vi "Read out  X Sensor.vi"() -> (1 "error out":errorcluster, 2 "Result":dbl format="%#_5p")   [LabVIEW 2013]
panel:
  # "Read Out XSensor"
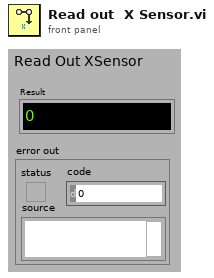
[diagram p1: front panel]
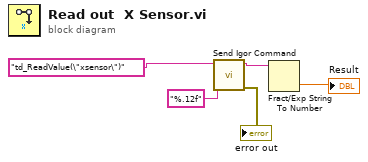
[diagram p0: block diagram]
diagram:
  n1 = call "Send Igor Command.vi"("Command"="td_ReadValue(\"xsensor\")", "Expected output Format"="%.12f") -> ("results"=w3:string, "error out"=→"error out":errorcluster)  [unwired: 6 in, 1 out]
  n2 = Fract/Exp String To Number(string=w3) -> (number=→"Result":dbl)  [unwired: 4 out]
